vi "Voltage - Finite Input.vi"() -> ()   [LabVIEW 2021]
doc: "This example demonstrates how to acquire a single buffer of voltage measurements using a DAQmx device.\n\nFor instructions on how to connect your signals to the DAQ device, refer to your device documentation."
uses:
  <vilib>/Utility/error.llb/DialogType.ctl
  <vilib>/DAQmx/read.llb/DAQmx Read (Analog 1D Wfm NChan NSamp).vi
  <vilib>/DAQmx/create/channels.llb/DAQmx Create Channel (AI-Voltage-Basic).vi
  <vilib>/DAQmx/configure/timing.llb/DAQmx Timing (Sample Clock).vi
  <vilib>/DAQmx/configure/task.llb/DAQmx Configure Logging (TDMS).vi
  <vilib>/DAQmx/configure/trigger.llb/DAQmx Start Trigger (Digital Edge).vi
  <vilib>/DAQmx/configure/trigger.llb/DAQmx Start Trigger (Time).vi
  <vilib>/DAQmx/configure/trigger.llb/DAQmx Start Trigger (Analog Edge).vi
  <vilib>/DAQmx/configure/trigger.llb/DAQmx Reference Trigger (Digital Edge).vi
  <vilib>/DAQmx/configure/trigger.llb/DAQmx Reference Trigger (Analog Edge).vi
  <vilib>/DAQmx/miscellaneous.llb/DAQmx Fill In Error Info.vi
  <resource>/objmgr/daqmx.rc
panel:
  in  "Trigger Type":T1(tab)
  in  "Digital Start Trigger Edge":i32(ring)=10280 caption="Edge" items=["Rising"=10280, "Falling"=10171]
  in  "Digital Start Trigger Source":tag="/Dev1/PFI0" caption="Source"
  in  "Digital Pause Trigger Pause When":i32(ring)=10192 caption="Pause When" items=["High"=10192, "Low"=10214]
  in  "Digital Pause Trigger Source":tag="/Dev1/PFI0" caption="Source"
  in  "Digital Reference Trigger Source":tag="/Dev1/PFI0" caption="Source"
  in  "Digital Reference Trigger Edge":i32(ring)=10280 caption="Edge" items=["Rising"=10280, "Falling"=10171]
  in  "Digital Reference Pretrigger Samples":u32 caption="Pretrigger Samples"
  in  "Analog Start Trigger Level":dbl caption="Level" format="%0.2f"
  in  "Analog Start Trigger Hysteresis":dbl caption="Hysteresis" format="%.2f"
  in  "Analog Start Trigger Slope":i32(ring)=10280 caption="Slope" items=["Rising"=10280, "Falling"=10171]
  in  "Analog Start Trigger Source":string="APFI0" caption="Source"
  in  "Analog Pause Trigger Source":string="APFI0" caption="Source"
  in  "Analog Pause Trigger Pause When":i32(ring)=10093 caption="Pause When" items=["Above Level"=10093, "Below Level"=10107]
  in  "Analog Pause Trigger Level":dbl caption="Level" format="%.2f"
  in  "Analog Reference Trigger Source":string="APFI0" caption="Source"
  in  "Analog Reference Trigger Level":dbl caption="Level" format="%.2f"
  in  "Analog Reference Trigger Slope":i32(ring)=10280 caption="Slope" items=["Rising"=10280, "Falling"=10171]
  in  "Analog Reference Pretrigger Samples":u32 caption="Pretrigger Samples"
  in  "When":timestamp
  in  "Select Time\nManually":bool
  out "Waveform Graph":waveform(dbl)[](graph)
  in  "TDMS File Path":path
  in  "Number of Samples":i32=100
  in  "Sample Rate":dbl=1000.0
  in  "Sample Clock Source":tag="OnboardClock"
  in  "Terminal Configuration":i32(ring)=-1 items=["default"=-1, "RSE"=10083, "NRSE"=10078, "Differential"=10106, "Pseudodifferential"=12529]
  in  "Max Voltage":dbl=5.0
  in  "Min Voltage":dbl=-5.0
  in  "Physical Channel":tag="PXI2Slot2/ai0"
  out "Actual Sample Rate":dbl=1000.0 format="%0.2f"
  in  "Logging Mode":i32(ring)=10231 items=["Off"=10231, "Log and Read"=15842]
  # "Channel Settings"
  # "Acquired Data"
  # "Timing Settings"
  # "Trigger Settings"
  # "Logging Settings"
  # "To enable triggers, select a tab above, and configure the settings.\n\nNot all hardware supports all trigger types. Refer to your device documentation for more information."
  # "If time is not manually set, task will begin after 10 seconds"
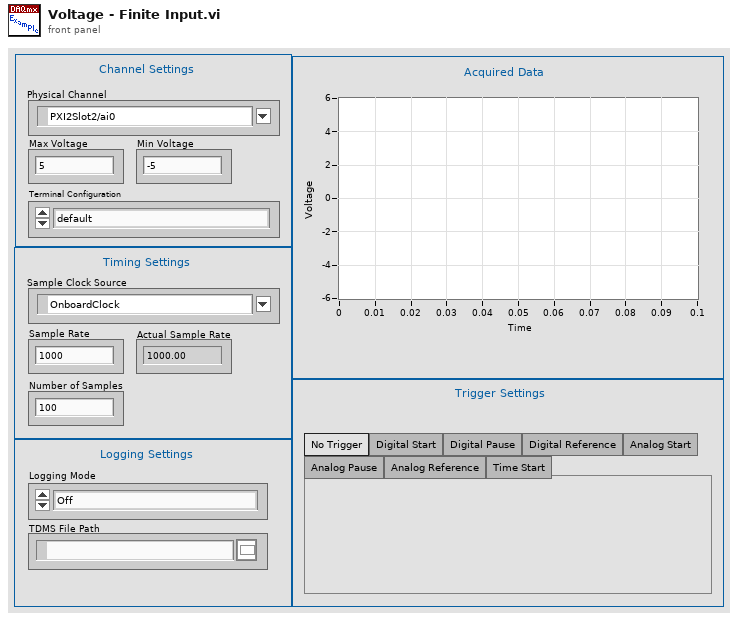
[diagram p1: front panel]
types:
  T1 = enum32{"No Trigger", "Digital Start", "Digital Pause", "Digital Reference", "Analog Start", "Analog Pause", "Analog Reference", "Time Start"}
  T2 = typedef "DialogType.ctl" = u16
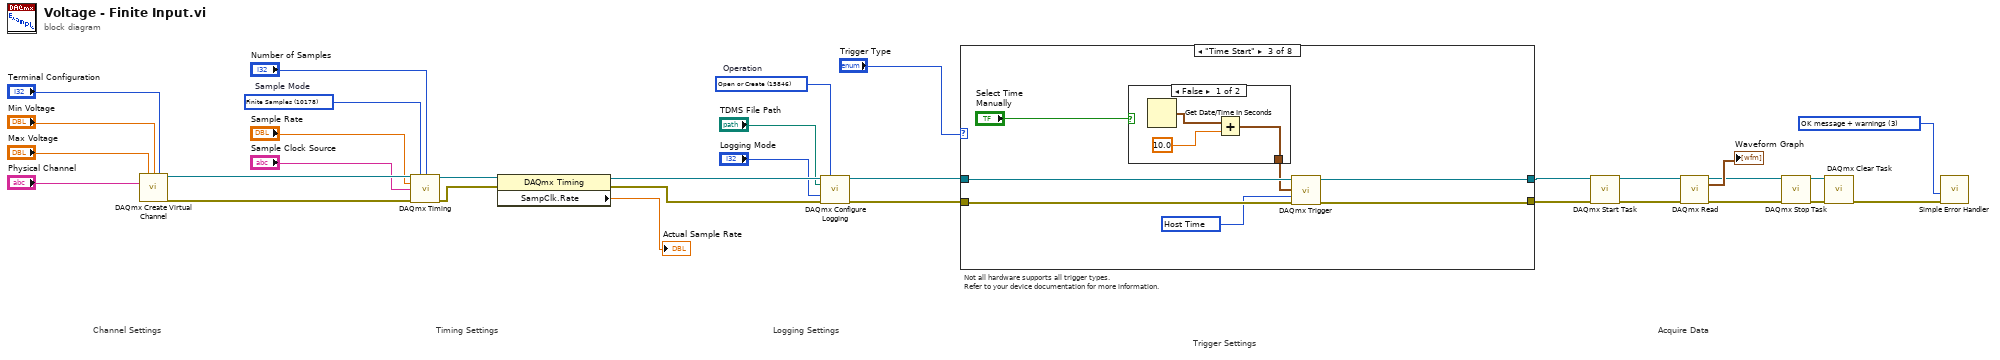
[diagram p0: block diagram]
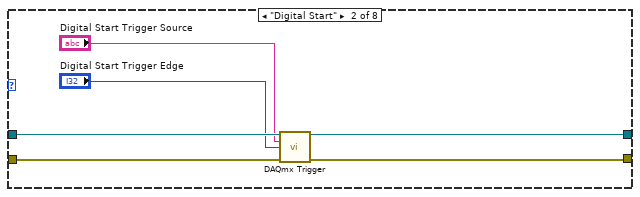
[diagram p3: hidden frame]
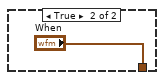
[diagram p4: hidden frame]
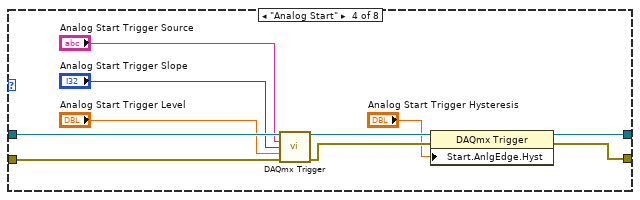
[diagram p5: hidden frame]
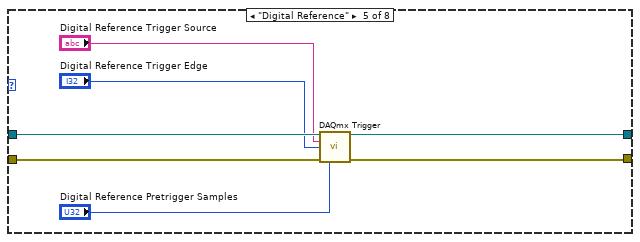
[diagram p6: hidden frame]
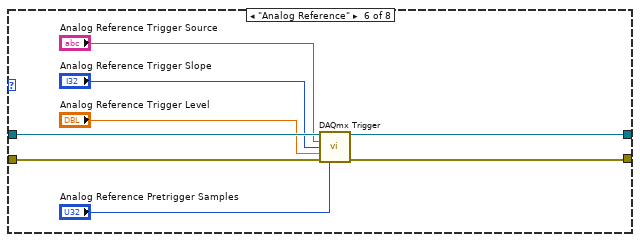
[diagram p7: hidden frame]
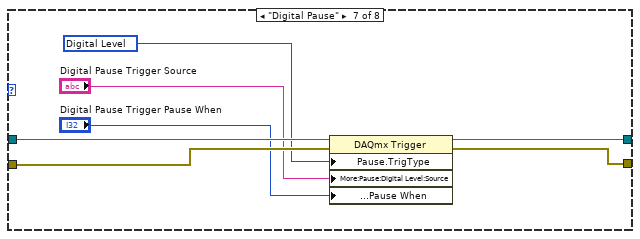
[diagram p8: hidden frame]
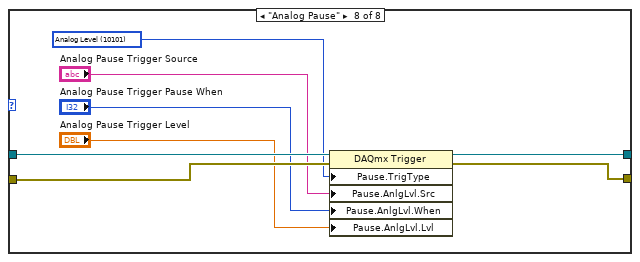
[diagram p9: hidden frame]
diagram:
  w6 = T2 3 items=["no dialog", "OK message", "continue or stop message", "OK message + warnings", "continue/stop + warnings"] ("type of dialog (OK msg:1)")
  w25 = 15846 items=["Open"=10437, "Open or Create"=15846, "Create or Replace"=15847, "Create"=15848]  # Operation
  w30 = 10178 items=["Finite Samples"=10178, "Continuous Samples"=10123, "Hardware Timed Single Point"=12522]  # Sample Mode
  # "Not all hardware supports all trigger types.\nRefer to your device documentation for more information."
  # "Trigger Settings"
  # "Acquire Data"
  # "Timing Settings"
  # "Channel Settings"
  # "Logging Settings"
  n1 = call-poly <vilib>:"DAQmx Create Virtual Channel.vi"("maximum value"="Max Voltage", "minimum value"="Min Voltage", "input terminal configuration"="Terminal Configuration", "physical channels"="Physical Channel") -> ("task out"=w28:refnum<k21>, "error out"=w29:errorcluster)  [unwired: 10 in]
  n2 = call-poly <vilib>:"DAQmx Timing.vi"("task/channels in"=w28, "sample mode"=w30, "samples per channel"="Number of Samples", "rate"="Sample Rate", "source"="Sample Clock Source", "error in"=w29) -> ("task out"=w32:refnum<k21>, "error out"=w31:errorcluster)  [unwired: 8 in]
  n3 = property class="DAQmx Timing"(reference=w32, error in=w31) -> (reference out=w27:refnum<k21>, error out=w26:errorcluster, "SampClk.Rate"=→"Actual Sample Rate":dbl)
  n4 = call-poly <vilib>:"DAQmx Configure Logging.vi"("task/channels in"=w27, "operation"=w25, "file path"="TDMS File Path", "logging mode"="Logging Mode", "error in"=w26) -> ("task out"=w4:refnum<k21>, "error out"=w3:errorcluster)  [unwired: 9 in]
  n5 = case shown="\"Time Start\"" "Trigger Type" {
    tunnel: w4 -> [w34 w40 w47 w61 w68 w76 w83 w91]
    tunnel: w3 -> [w33 w39 w46 w60 w67 w75 w80 w88]
    tunnel: [w34 w38 w45 w58 w66 w74 w82 w90] -> w2
    tunnel: [w33 w37 w44 w57 w65 w73 w81 w89] -> w1
    frame "No Trigger", Default {
    }
    frame "Digital Start" {
      n6 = call-poly <vilib>:"DAQmx Trigger.vi"("task/channels in"=w40, "source"="Digital Start Trigger Source", "edge"="Digital Start Trigger Edge", "error in"=w39) -> ("task out"=w38:refnum<k21>, "error out"=w37:errorcluster)  [unwired: 10 in]
    }
    frame "Time Start" {
      w43 = 16126 items=["Host Time"=16126, "I/O Device Time"=16127] ("timescale")
      n7 = case shown="False" "Select Time\nManually" {
        tunnel: [w49 "When"] -> w41
        frame False {
          n8 = Get Date/Time In Seconds() -> (seconds since 1Jan1904=w50:timestamp)
          n9 = Add(x=w50, y=10.0) -> (x+y=w49:timestamp)
        }
        frame True {
        }
      }
      n10 = call-poly <vilib>:"DAQmx Trigger.vi"("task/channels in"=w47, "when"=w41, "timescale"=w43, "error in"=w46) -> ("task out"=w45:refnum<k21>, "error out"=w44:errorcluster)  [unwired: 10 in]
    }
    frame "Analog Start" {
      n11 = call-poly <vilib>:"DAQmx Trigger.vi"("task/channels in"=w61, "source"="Analog Start Trigger Source", "slope"="Analog Start Trigger Slope", "level"="Analog Start Trigger Level", "error in"=w60) -> ("task out"=w56:refnum<k21>, "error out"=w55:errorcluster)  [unwired: 9 in]
      n12 = property class="DAQmx Trigger"(reference=w56, error in=w55, "Start.AnlgEdge.Hyst"="Analog Start Trigger Hysteresis") -> (reference out=w58:refnum<k21>, error out=w57:errorcluster)
    }
    frame "Digital Reference" {
      n13 = call-poly <vilib>:"DAQmx Trigger.vi"("task/channels in"=w68, "source"="Digital Reference Trigger Source", "edge"="Digital Reference Trigger Edge", "error in"=w67, "pretrigger samples per channel"="Digital Reference Pretrigger Samples") -> ("task out"=w66:refnum<k21>, "error out"=w65:errorcluster)  [unwired: 9 in]
    }
    frame "Analog Reference" {
      n14 = call-poly <vilib>:"DAQmx Trigger.vi"("task/channels in"=w76, "source"="Analog Reference Trigger Source", "slope"="Analog Reference Trigger Slope", "level"="Analog Reference Trigger Level", "error in"=w75, "pretrigger samples per channel"="Analog Reference Pretrigger Samples") -> ("task out"=w74:refnum<k21>, "error out"=w73:errorcluster)  [unwired: 8 in]
    }
    frame "Digital Pause" {
      w79 = 10152 items=["Analog Level"=10101, "Analog Window"=10103, "Digital Level"=10152, "Digital Pattern"=10398, "None"=10230] ("Pause.TrigType")
      n15 = property class="DAQmx Trigger"(reference=w83, error in=w80, "Pause.TrigType"=w79, "More:Pause:Digital Level:Source"="Digital Pause Trigger Source", "More:Pause:Digital Level:Pause When"="Digital Pause Trigger Pause When") -> (reference out=w82:refnum<k21>, error out=w81:errorcluster)
    }
    frame "Analog Pause" {
      w87 = 10101 items=["Analog Level"=10101, "Analog Window"=10103, "Digital Level"=10152, "Digital Pattern"=10398, "None"=10230] ("Pause.TrigType")
      n16 = property class="DAQmx Trigger"(reference=w91, error in=w88, "Pause.TrigType"=w87, "Pause.AnlgLvl.Src"="Analog Pause Trigger Source", "Pause.AnlgLvl.When"="Analog Pause Trigger Pause When", "Pause.AnlgLvl.Lvl"="Analog Pause Trigger Level") -> (reference out=w90:refnum<k21>, error out=w89:errorcluster)
    }
  }
  n17 = call <vilib>:"DAQmx Start Task.vi"("task/channels in"=w2, "error in"=w1) -> ("task out"=w24:refnum<k21>, "error out"=w23:errorcluster)  [unwired: 12 in]
  n18 = call-poly <vilib>:"DAQmx Read.vi"("task/channels in"=w24, "error in"=w23) -> ("task out"=w8:refnum<k21>, "data"=→"Waveform Graph":waveform(dbl)[], "error out"=w7:errorcluster)  [unwired: 11 in]
  n19 = call <vilib>:"DAQmx Stop Task.vi"("task/channels in"=w8, "error in"=w7) -> ("task out"=w10:refnum<k21>, "error out"=w9:errorcluster)  [unwired: 12 in]
  n20 = call <vilib>:"DAQmx Clear Task.vi"("task in"=w10, "error in"=w9) -> ("error out"=w22:errorcluster)  [unwired: 13 in]
  n21 = call <vilib>:"Simple Error Handler.vi"("type of dialog (OK msg:1)"=w6, "error in (no error)"=w22) -> ()  [unwired: 3 in, 5 out]
